vi "DestroySurface.vi"(8 "No Error":errorcluster, 11 "Surface [SDL_Surface *]":i64 format="%.0x") -> (0 "error out":errorcluster)   [LabVIEW 2024, in "SDL3.lvlib" / "Surface.lvlib"]
doc: "<B>Summary</B>\nFree a surface.\n\n<B>Remarks</B>\nIt is safe to pass NULL to this function."
uses:
  Surface.lvlib
  Lib/Win32/SDL3.dll
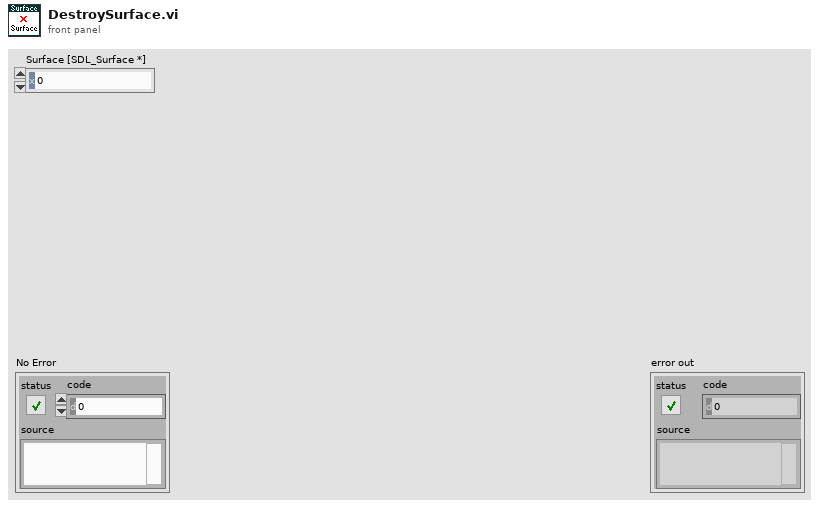
[diagram p1: front panel]
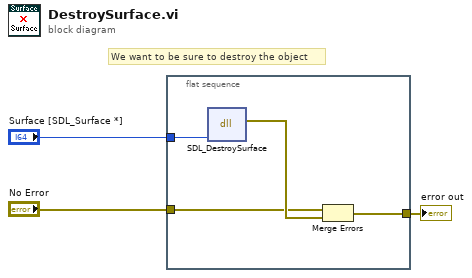
[diagram p0: block diagram]
diagram:
  # "We want to be sure to destroy the object"
  n1 = flat-sequence {
    tunnel: [w6] -> w3
    tunnel: "No Error" -> [w5]
    tunnel: "Surface [SDL_Surface *]" -> [w4]
    frame #0 {
      n2 = dll-call lib="C:/Users/Thomas/Documents/Projects/LV-SDL3/Lib/Win32/SDL3.dll" fn="SDL_DestroySurface"("surface"=w4) -> (error out=w7:errorcluster)  [unwired: 5 in, 1 out]
      n3 = Merge Errors(w5, w7) -> (w6:errorcluster)
    }
  }
  "error out" <- w3
